vi "SSL_Check.vi"(8 "error in (no error)":errorcluster, 9 "Barcode_Can_Read":string, 10 "Section":string, 11 "instrument file path":path) -> (0 "error out":errorcluster, 3 "RX/RY":string)   [LabVIEW 2024]
uses:
  <vilib>/Utility/file.llb/Read Delimited Spreadsheet (string).vi
  Launcher/Launcher_DTU.lvlib
panel:
  out "Barcode_Column":string[](array[string])
  out "Csv_File":string[][](array[string])
  out "element":string
  out "Values out":string[](array[string])
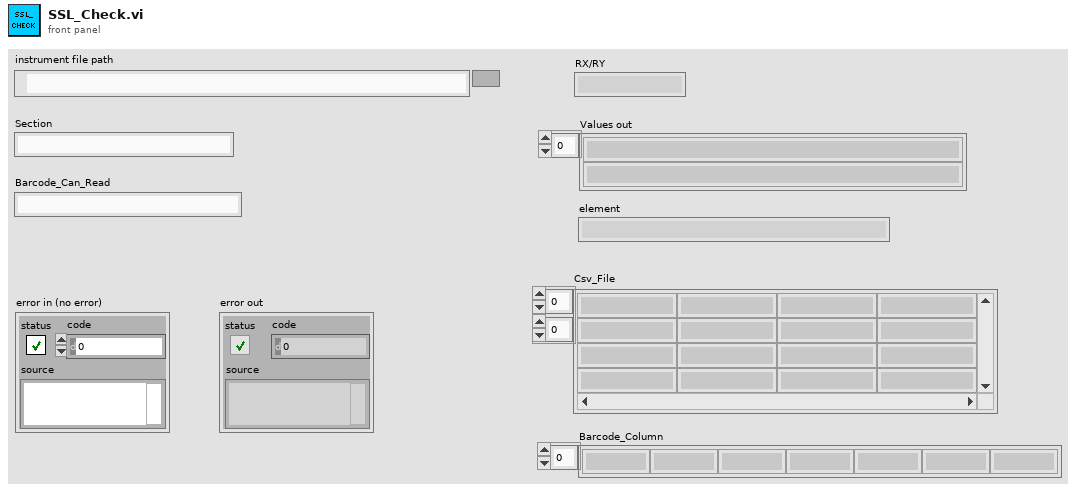
[diagram p1: front panel]
types:
  T1 = enum16{"Read", "Write", "All_sections", "All_values", "Remove key&section"}
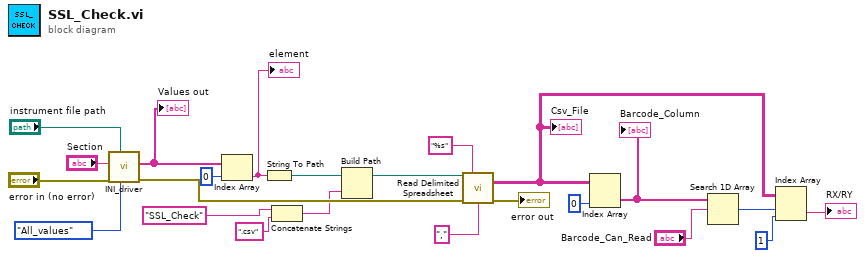
[diagram p0: block diagram]
diagram:
  n1 = call "INI_driver.vi"("Enum"=T1."All_values", "instrument file path"="instrument file path", "error in (no error)"="error in (no error)", "Section"="Section") -> ("error out"=w13:errorcluster, "Values out"=w20:string[])  [unwired: 4 in, 2 out]
  "Values out" <- w20
  n2 = Index Array(array=w20, index=0) -> (element=w18:string)
  "element" <- w18
  n3 = String To Path(string=w18) -> (path=w16:path)
  n4 = Concatenate Strings("SSL_Check" ("string"), ".csv" ("string")) -> (w2:string)
  n5 = Build Path(base path=w16, name or relative path=w2) -> (appended path=w4:path)
  n6 = call-poly <vilib>:"Read Delimited Spreadsheet.vi"("file path (dialog if empty)"=w4, "format (%s)"="%s", "error in (no error)"=w13, "delimiter (\\t)"="," ("delimiter (\\t)")) -> ("all rows"=w8:string[][], "error out"=→"error out":errorcluster)  [unwired: 6 in, 4 out]
  "Csv_File" <- w8
  n7 = Index Array(array=w8, index (col)=0 ("disabled index (col)")) -> (element=w11:string[])  [unwired: 1 in]
  "Barcode_Column" <- w11
  n8 = Search 1D Array(1D array=w11, element="Barcode_Can_Read") -> (index of element=w9:i32)  [unwired: 1 in]
  n9 = Index Array(array=w8, index (row)=w9, index (col)=1 ("disabled index (col)")) -> (element=→"RX/RY":string)
